vi "Read Steps.vi"(8 "error in (no error)":errorcluster, 11 "Parallel Step in":refnum<class "Parallel Step.lvclass">) -> (0 "error out":errorcluster, 2 "Steps":refnum<class "Step.lvclass">[](array[class]), 3 "Parallel Step out":refnum<class "Parallel Step.lvclass">)   [LabVIEW 2015, in "Parallel Step.lvclass"]
uses:
  Parallel Step.lvclass
  classes/Step/Execution/Step.lvclass
  Parallel Step.lvclass/Parallel Step.ctl
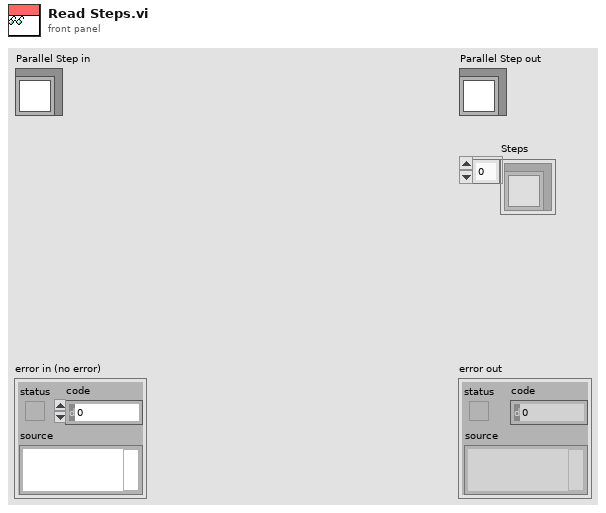
[diagram p1: front panel]
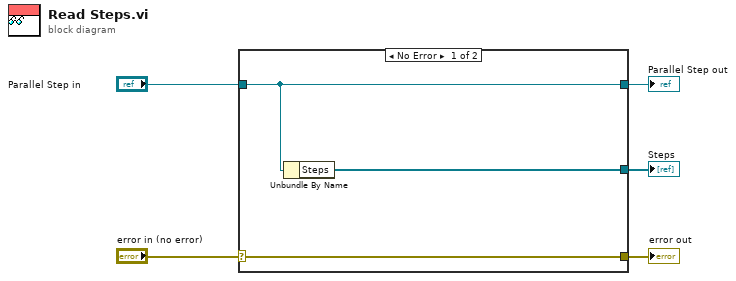
[diagram p0: block diagram]
diagram:
  n1 = case shown="No Error" "error in (no error)" {
    selector: "error in (no error)" -> [w8 w9]
    tunnel: [w8 w9] -> w4
    tunnel: [w7 w10] -> w2
    tunnel: "Parallel Step in" -> [w7 w10]
    tunnel: [w6 _] -> w1
    frame No Error {
      n2 = Unbundle By Name(w7) -> ("Steps"=w6:refnum<class "Step.lvclass">[])
    }
    frame Error {
    }
  }
  "error out" <- w4
  "Parallel Step out" <- w2
  "Steps" <- w1
